vi "Refresh References.vi"(8 "error in (no error)":errorcluster, 11 "CSM-Helper in":refnum<class "CSM-Helper.lvclass">) -> (0 "error out":errorcluster, 3 "CSM-Helper out":refnum<class "CSM-Helper.lvclass">)   [LabVIEW 2020, in "CSM-Helper.lvclass"]
uses:
  CSM-Helper.lvclass
  CSM-Helper.lvclass/CSM-Helper.ctl
  <vilib>/Utility/Data Type/Type Definitions/Data Type.ctl
  <vilib>/Utility/Data Type/Type Definitions/Refnum Type.ctl
  <vilib>/Utility/Data Type/NI_Data Type.lvlib
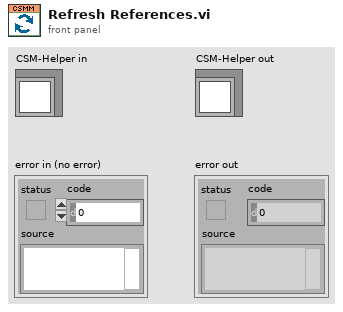
[diagram p1: front panel]
types:
  T1 = cluster{refnum<vi>, "Outer Term":refnum<vi>, "Data Type":variant, "Wire":refnum<vi>}
  T2 = typedef "NI_Data Type.lvlib/Data Type.ctl" = enum8{"Invalid Type", "Void", "I8", "I16", "I32", "I64", "U8", "U16", "U32", "U64", "Single Float", "Double Float", "Extended Float", "Single Complex", "Double Complex", "Extended Complex", "Enum U8", "Enum U16", "Enum U32", "Enum U64", "Single Float With Unit", "Double Float With Unit", "Extended Float With Unit", "Single Complex with Unit", "Double Complex with Unit", "Extended Complex with Unit", "Boolean", "String", "Path", "Picture", "Tag", "Array", "Cluster", "Variant", "LV Variant", "Waveform", "Timestamp", "Digital Waveform", "Digital Data", "ExpressData", "Refnum", "External Data", "VI", "Poly VI", "LabVIEW Class Instance", "Fixed Point", "Set Collection", "Map Collection"}
  T3 = typedef "NI_Data Type.lvlib/Type Definition Info.ctl" = cluster{"Name":string, "Timestamp":u32}
  T4 = typedef "NI_Data Type.lvlib/Refnum Type.ctl" = enum16{"NotARefnum", "UnknownRefnum", "Generic", "Datalog", "ByteStream", "Device", "Occurence", "TCPNetConnection", "Auto", "Menu", "Imaq", "Hardware", "DataSocket", "Visa", "IVI", "UDPNetConnection", "Notifier", "Queue", "Irda", "EventReg", "DotNet", "UserEvent", "Callback", "UNUSED_EMPTY_POSITION", "BlueToothNetConnection", "LVObjApp", "LVObjVI", "LVObjUnknown", "GenericClass", "UserDefinedRefnumTag", "DataValue", "RT FIFO", "TDMS File", "PythonSessionRefnum"}
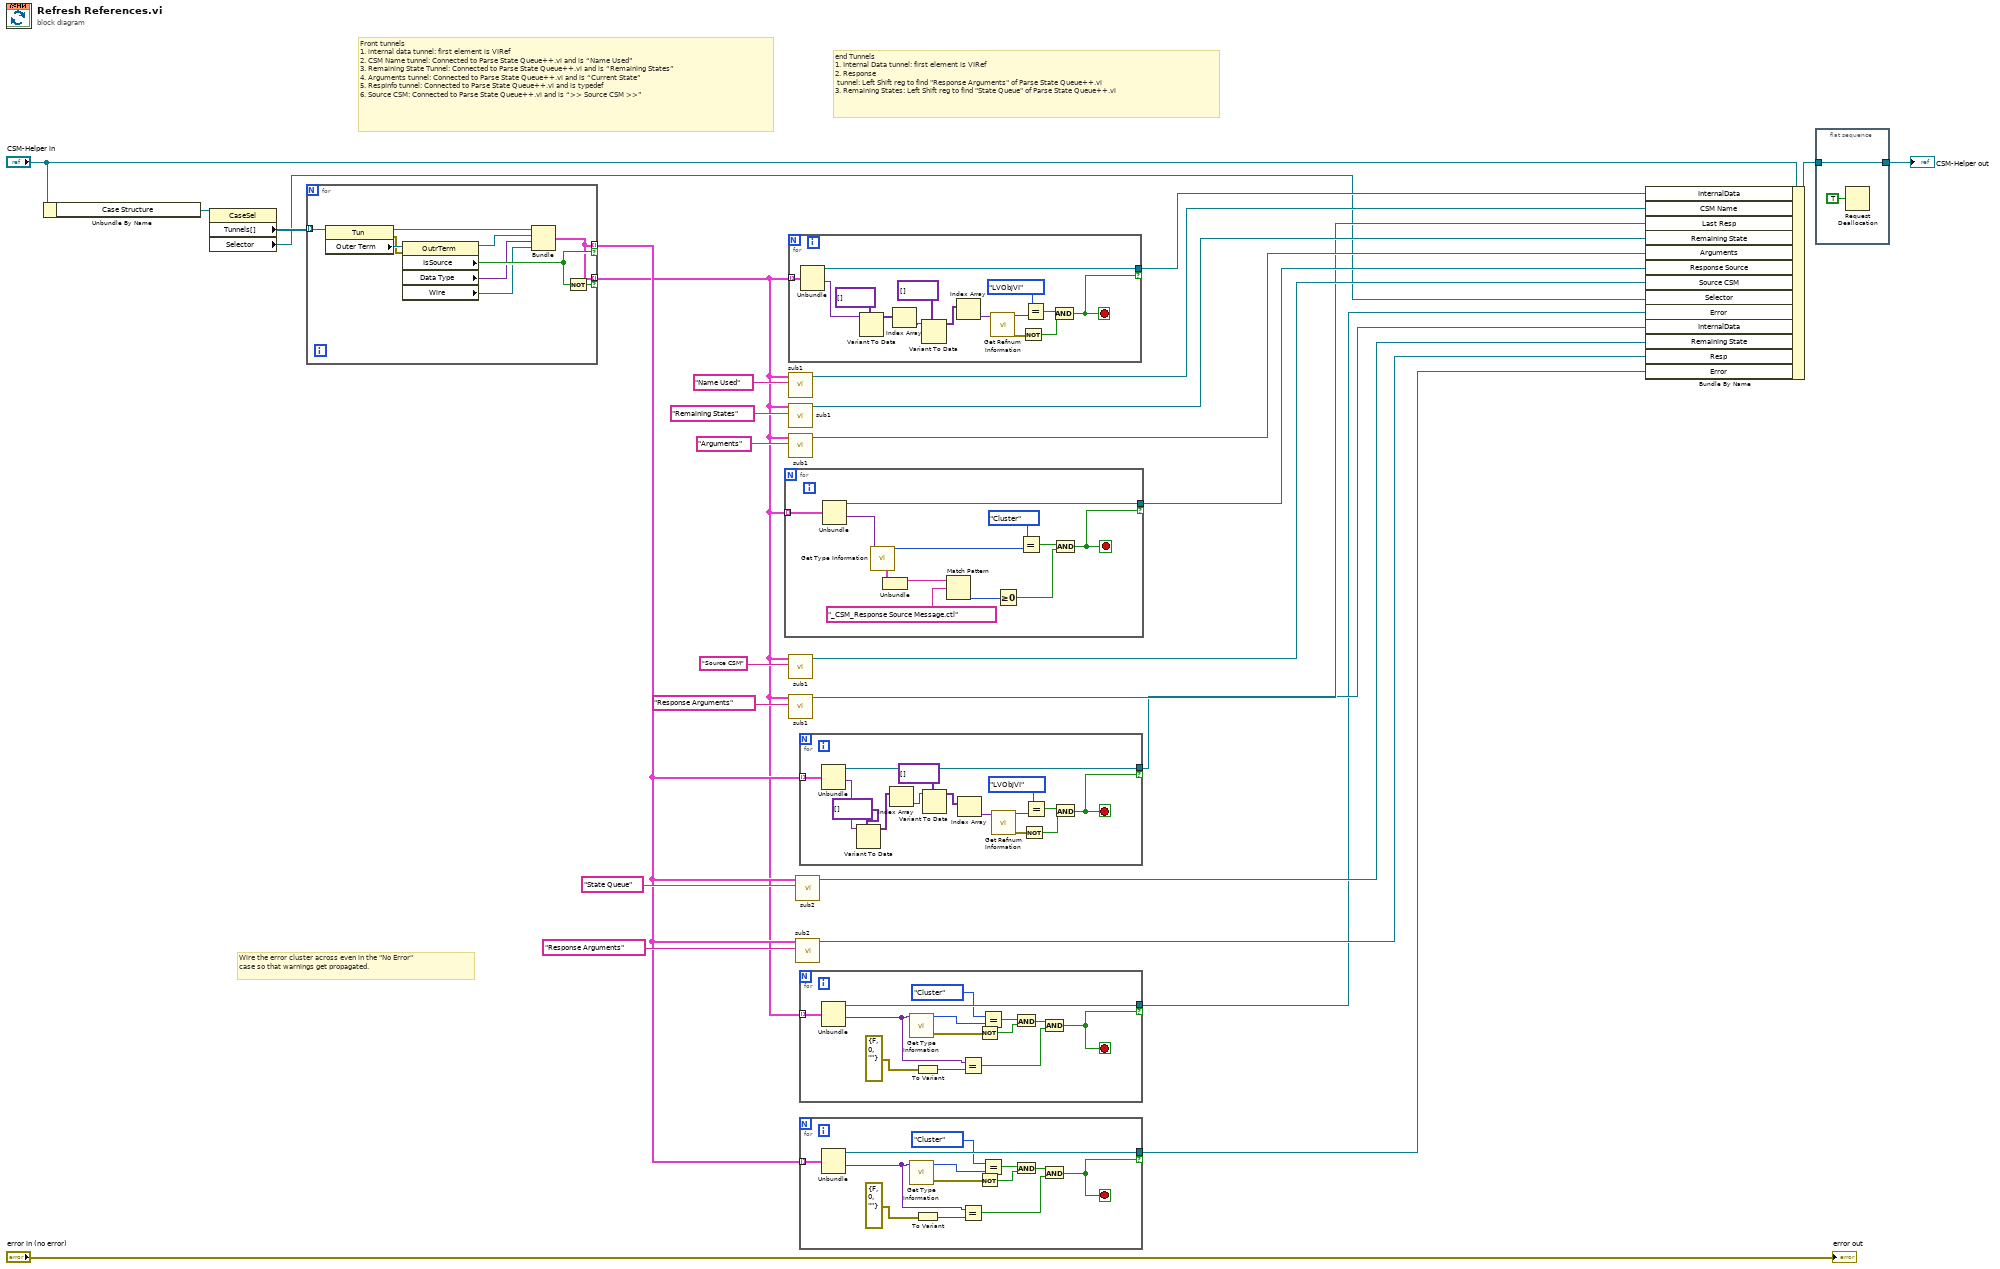
[diagram p0: block diagram]
diagram:
  # "end Tunnels\n1. Internal Data tunnel: first element is VIRef\n2. Response\n tunnel: Left Shift reg to find \"Response Arguments\" of Parse State Queue++.vi \n3. Remaining States: Left Shift reg to find \"State Queue\" of Parse State Queue++.vi"
  # "Front tunnels\n1. internal data tunnel: first element is VIRef\n2. CSM Name tunnel: Connected to Parse State Queue++.vi and is “Name Used”\n3. Remaining State Tunnel: Connected to Parse State Queue++.vi and is “Remaining States”\n4. Arguments tunnel: Connected to Parse State Queue++.vi and is “Current State”\n5. RespInfo tunnel: Connected to Parse State Queue++.vi and is typedef\n6. Source CSM: Connected to Parse State Queue++.vi and is “>> Source CSM >>”"
  # "Wire the error cluster across even in the \"No Error\"\ncase so that warnings get propagated."
  n1 = Unbundle By Name("CSM-Helper in") -> ("Case Structure"=w26:refnum<vi>)
  n2 = property class="CaseSel"(reference=w26) -> ("Tunnels[]"=w25:refnum<vi>[], "Selector"=w12:refnum<vi>)  [unwired: 1 in, 2 out]
  n3 = for {
    tunnel: w25 -> [w38] mode=indexing
    tunnel: [w31] -> w4 mode=indexing if=w35
    tunnel: [w31] -> w3 mode=indexing if=w34
    n4 = property class="Tun"(reference=w38) -> (reference out=w33:refnum<vi>, error out=w36:errorcluster, "Outer Term"=w37:refnum<vi>)  [unwired: 1 in]
    n5 = property class="OutrTerm"(reference=w37, error in=w36) -> (reference out=w32:refnum<vi>, "IsSource"=w35:bool, "Data Type"=w30:variant, "Wire"=w29:refnum<vi>)  [unwired: 1 out]
    n6 = Bundle(w33, "Outer Term"=w32, "Data Type"=w30, "Wire"=w29) -> (w31:T1)  [unwired: 1 in]
    n7 = Not(x=w35) -> (.not. x?=w34:bool)
  }
  n8 = for {
    tunnel: w3 -> [w50] mode=indexing
    tunnel: [w47] -> w15 if=w46
    stop <- w46 stop-if-true
    n9 = Unbundle(w50) -> (w47:refnum<vi>, "Data Type"=w43:variant)  [unwired: 2 out]
    n10 = call <vilib>:"Get Type Information.vi"("variant"=w43) -> ("type"=w49:T2, "type definition info"=w44:T3)  [unwired: 6 in, 3 out]
    n11 = Unbundle(w44) -> ("Name"=w42:string)  [unwired: 1 out]
    n12 = Match Pattern(string=w42, regular expression="_CSM_Response Source Message.ctl") -> (offset past match=w40:i32)  [unwired: 1 in, 3 out]
    n13 = Greater Or Equal To 0?(x=w40) -> (x >= 0?=w39:bool)
    n14 = Equal?(x=Data_Type."Cluster", y=w49) -> (x = y?=w48:bool)
    n15 = And(x=w48, y=w39) -> (x .and. y?=w46:bool)
  }
  n16 = for {
    tunnel: w3 -> [w65] mode=indexing
    tunnel: [w58] -> w24 if=w57
    stop <- w57 stop-if-true
    n17 = Unbundle(w65) -> (w58:refnum<vi>, "Data Type"=w55:variant)  [unwired: 2 out]
    n18 = Variant To Data(type=variant[] [] ("Array"), Variant=w55) -> (data=w54:variant[])  [unwired: 1 in, 1 out]
    n19 = Index Array(array=w54) -> (element=w52:variant)  [unwired: 1 in]
    n20 = Variant To Data(type=variant[] [] ("Array"), Variant=w52) -> (data=w51:variant[])  [unwired: 1 in, 1 out]
    n21 = Index Array(array=w51) -> (element=w64:variant)  [unwired: 1 in]
    n22 = call <vilib>:"Get Refnum Information.vi"("variant"=w64) -> ("error out"=w60:errorcluster, "reference type"=w62:T4)  [unwired: 7 in, 2 out]
    n23 = Not(x=w60) -> (.not. x?=w59:bool)
    n24 = Equal?(x=Refnum_Type."LVObjVI", y=w62) -> (x = y?=w61:bool)
    n25 = And(x=w61, y=w59) -> (x .and. y?=w57:bool)
  }
  n26 = call "sub1.vi"("regular expression"="Name Used", "Array"=w3) -> ("Tunnel out"=w23:refnum<vi>)  [unwired: 9 in]
  n27 = call "sub1.vi"("regular expression"="Remaining States", "Array"=w3) -> ("Tunnel out"=w20:refnum<vi>)  [unwired: 9 in]
  n28 = call "sub1.vi"("regular expression"="Arguments", "Array"=w3) -> ("Tunnel out"=w18:refnum<vi>)  [unwired: 9 in]
  n29 = call "sub1.vi"("regular expression"="Source CSM", "Array"=w3) -> ("Tunnel out"=w16:refnum<vi>)  [unwired: 9 in]
  n30 = call "sub1.vi"("regular expression"="Response Arguments", "Array"=w3) -> ("Tunnel out"=w13:refnum<vi>)  [unwired: 9 in]
  n31 = call "sub2.vi"("regular expression"="State Queue", "Array"=w4) -> ("Tunnel out"=w7:refnum<vi>)  [unwired: 9 in]
  n32 = call "sub2.vi"("regular expression"="Response Arguments", "Array"=w4) -> ("Tunnel out"=w5:refnum<vi>)  [unwired: 9 in]
  n33 = for {
    tunnel: w4 -> [w80] mode=indexing
    tunnel: [w73] -> w9 if=w72
    stop <- w72 stop-if-true
    n34 = Unbundle(w80) -> (w73:refnum<vi>, "Data Type"=w68:variant)  [unwired: 2 out]
    n35 = Variant To Data(type=variant[] [] ("Array"), Variant=w68) -> (data=w66:variant[])  [unwired: 1 in, 1 out]
    n36 = Index Array(array=w66) -> (element=w70:variant)  [unwired: 1 in]
    n37 = Variant To Data(type=variant[] [] ("Array"), Variant=w70) -> (data=w69:variant[])  [unwired: 1 in, 1 out]
    n38 = Index Array(array=w69) -> (element=w79:variant)  [unwired: 1 in]
    n39 = call <vilib>:"Get Refnum Information.vi"("variant"=w79) -> ("error out"=w75:errorcluster, "reference type"=w77:T4)  [unwired: 7 in, 2 out]
    n40 = Not(x=w75) -> (.not. x?=w74:bool)
    n41 = Equal?(x=Refnum_Type."LVObjVI", y=w77) -> (x = y?=w76:bool)
    n42 = And(x=w76, y=w74) -> (x .and. y?=w72:bool)
  }
  n43 = for {
    tunnel: w3 -> [w93] mode=indexing
    tunnel: [w92] -> w2 if=w81
    stop <- w81 stop-if-true
    n44 = Unbundle(w93) -> (w92:refnum<vi>, "Data Type"=w88:variant)  [unwired: 2 out]
    n45 = call <vilib>:"Get Type Information.vi"("variant"=w88) -> ("error out"=w89:errorcluster, "type"=w91:T2)  [unwired: 6 in, 3 out]
    n46 = To Variant(anything=errorcluster {"status"=FALSE, "code"=0, "source"=""} ("error in (no error)")) -> (Variant=w86:variant)
    n47 = Equal?(x=w88, y=w86) -> (x = y?=w82:bool)
    n48 = Not(x=w89) -> (.not. x?=w84:bool)
    n49 = Equal?(x=Data_Type."Cluster", y=w91) -> (x = y?=w85:bool)
    n50 = And(x=w85, y=w84) -> (x .and. y?=w83:bool)
    n51 = And(x=w83, y=w82) -> (x .and. y?=w81:bool)
  }
  n52 = for {
    tunnel: w4 -> [w106] mode=indexing
    tunnel: [w105] -> w1 if=w94
    stop <- w94 stop-if-true
    n53 = Unbundle(w106) -> (w105:refnum<vi>, "Data Type"=w101:variant)  [unwired: 2 out]
    n54 = call <vilib>:"Get Type Information.vi"("variant"=w101) -> ("error out"=w102:errorcluster, "type"=w104:T2)  [unwired: 6 in, 3 out]
    n55 = To Variant(anything=errorcluster {"status"=FALSE, "code"=0, "source"=""} ("error in (no error)")) -> (Variant=w99:variant)
    n56 = Equal?(x=w101, y=w99) -> (x = y?=w95:bool)
    n57 = Not(x=w102) -> (.not. x?=w97:bool)
    n58 = Equal?(x=Data_Type."Cluster", y=w104) -> (x = y?=w98:bool)
    n59 = And(x=w98, y=w97) -> (x .and. y?=w96:bool)
    n60 = And(x=w96, y=w95) -> (x .and. y?=w94:bool)
  }
  n61 = Bundle By Name(cluster="CSM-Helper in", "InternalData"=w24, "CSM Name"=w23, "Last Resp"=w13, "Remaining State"=w20, "Arguments"=w18, "Response Source"=w15, "Source CSM"=w16, "Selector"=w12, "Error"=w2, "InternalData"=w9, "Remaining State"=w7, "Resp"=w5, "Error"=w1) -> (w11:refnum<class "CSM-Helper.lvclass">)
  n62 = flat-sequence {
    tunnel: w11 -> [w107]
    tunnel: [w107] -> w10
    frame #0 {
      n63 = Request Deallocation(TRUE ("flag")) -> ()
    }
  }
  "error out" <- "error in (no error)"
  "CSM-Helper out" <- w10
